vi "Next Message (No Metrics).vi"(8 "error in (no error)":errorcluster, 9 "Timeout ms (-1)":i32=-1, 11 "Module in":refnum<class "Module.lvclass">) -> (0 "error out":errorcluster, 1 "Data":variant, 2 "ID":string, 3 "Module out":refnum<class "Module.lvclass">)   [LabVIEW 2020, in "Volatus.lvlib" / "Module.lvclass"]
uses:
  Module.lvclass
  Module.lvclass/Module.ctl
  MessageQ/MessageQ.lvclass/MessageQ.ctl
  Module Status Update.ctl
  MessageQ/MessageQ.lvclass
  State.ctl
  Module Substatus.ctl
  Metric Update.ctl
  Launch Nested Message.ctl
  VolatusConfig/VolatusConfigElement/VolatusConfigElement.lvclass
  LastAck.ctl
  Update Metric.vi
  Parent Q.vi
  MessageQ/Is Null.vi
  MessageQ/Send.vi
  Volatus.lvlib
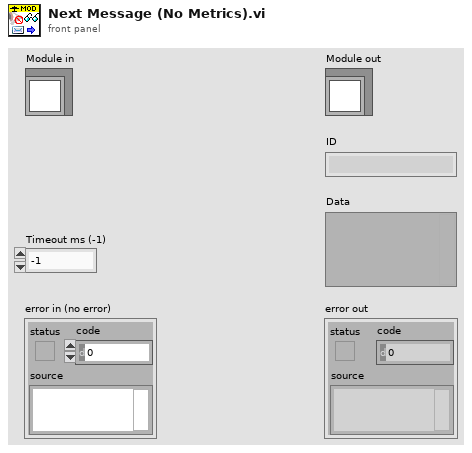
[diagram p1: front panel]
types:
  T1 = typedef "Volatus.lvlib/Module Status Update.ctl" = cluster{"MessageQ":refnum<class "MessageQ.lvclass">, "State":T2, "Hierarchy":string[], "Forwarded":bool}
  T2 = typedef "Volatus.lvlib/Module.lvclass/State.ctl" = enum16{"Unknown", "Launched", "Starting", "Running", "Stopping", "Stopped", "Error - Starting", "Error - Run", "Error - Stopping"}
  T3 = typedef "Volatus.lvlib/Module Substatus.ctl" = cluster{"Hierarchy":string[], "Name":string, "Status":string}
  T4 = typedef "Volatus.lvlib/Metric Update.ctl" = cluster{"Hierarchy":string[], "Name":string, "Value":dbl}
  T5 = typedef "Volatus.lvlib/Launch Nested Message.ctl" = cluster{"Module":refnum<class "Module.lvclass">, "Config":refnum<class "VolatusConfigElement.lvclass">}
  T6 = typedef "Volatus.lvlib/Module.lvclass/LastAck.ctl" = cluster{"Module":refnum<class "Module.lvclass">}
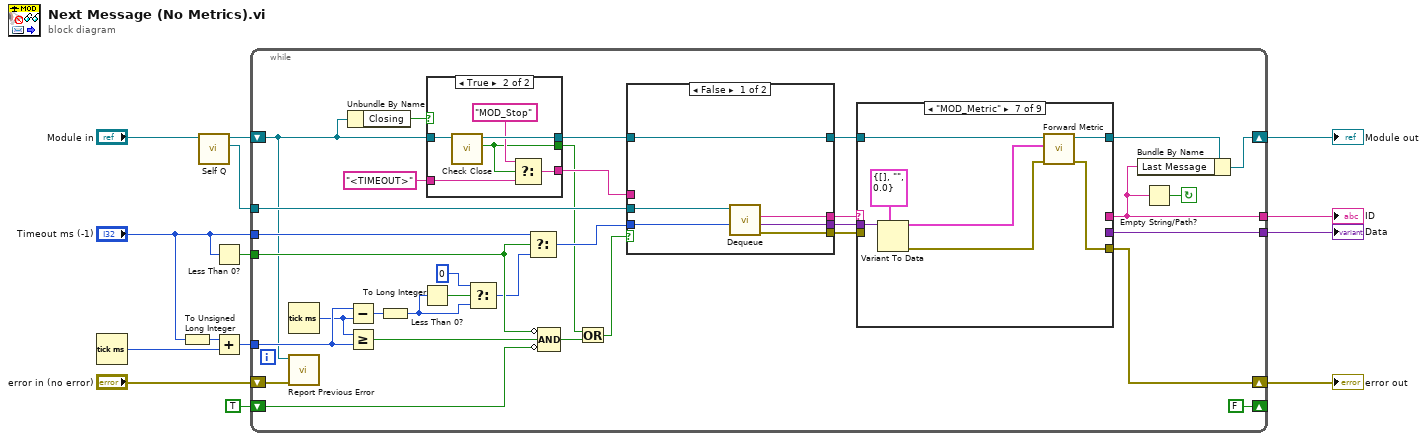
[diagram p0: block diagram]
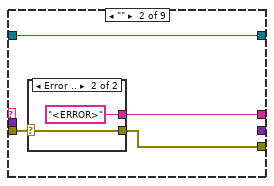
[diagram p5: hidden frame]
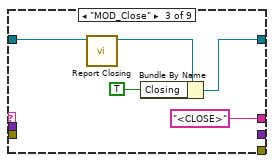
[diagram p7: hidden frame]
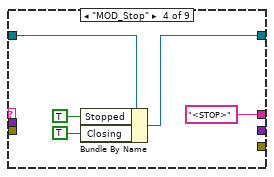
[diagram p8: hidden frame]
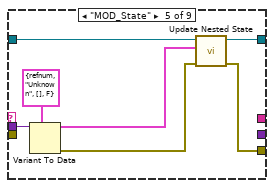
[diagram p9: hidden frame]
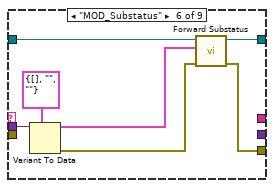
[diagram p10: hidden frame]
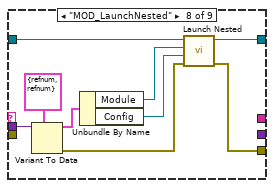
[diagram p11: hidden frame]
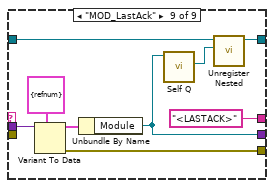
[diagram p12: hidden frame]
diagram:
  n1 = Tick Count (ms)() -> (millisecond timer value=w11:u32)
  n2 = To Unsigned Long Integer(number="Timeout ms (-1)") -> (unsigned 32bit integer=w10:u32)
  n3 = call "Self Q.vi"("Module in"="Module in") -> ("Self Q"=w12:refnum<class "MessageQ.lvclass">, "Module out"=w13:refnum<class "Module.lvclass">)  [unwired: 9 in]
  n4 = Less Than 0?(x="Timeout ms (-1)") -> (x < 0?=w6:bool)
  n5 = Add(x=w10, y=w11) -> (x+y=w9:u32)
  n6 = while {
    shift-right: [w31] -> w1
    shift-left: w13 -> [w15]
    tunnel: w12 -> [w46]
    tunnel: w9 -> [w37]
    tunnel: [w33] -> w3
    tunnel: [w41] -> w8
    tunnel: "Timeout ms (-1)" -> [w39]
    tunnel: w6 -> [w29]
    shift-right: [w34] -> w4
    shift-left: "error in (no error)" -> [w47]
    shift-right: [FALSE] -> _
    shift-left: TRUE -> [w27]
    stop <- w40 continue-if-true
    n7 = Tick Count (ms)() -> (millisecond timer value=w36:u32)
    n8 = call "Report Previous Error.vi"("error in (no error)"=w47, "Module in"=w15) -> ()  [unwired: 8 in, 2 out]
    n9 = Unbundle By Name(w15) -> ("Closing"=w22:bool)
    n10 = Subtract(x=w37, y=w36) -> (x-y=w45:u32)
    n11 = Greater Or Equal?(x=w36, y=w37) -> (x >= y?=w35:bool)
    n12 = To Long Integer(number=w45) -> (32bit integer=w24:i32)
    n13 = Less Than 0?(x=w24) -> (x < 0?=w26:bool)
    n14 = case shown="True" w22 {
      tunnel: w15 -> [w49 w55]
      tunnel: [w49 w54] -> w17
      tunnel: "<TIMEOUT>" ("ID") -> [w48 w53]
      tunnel: [w48 w51] -> w20
      tunnel: [_ w50] -> w18
      frame False {
      }
      frame True {
        n15 = call "Check Close.vi"("Module in"=w55) -> ("Stop"=w50:bool, "Module out"=w54:refnum<class "Module.lvclass">)  [unwired: 8 in, 1 out]
        n16 = Select(t="MOD_Stop", s=w50, f=w53) -> (s? t:f=w51:string)
      }
    }
    n17 = Select(t=0 ("32bit integer"), s=w26, f=w24) -> (s? t:f=w23:i32)
    n18 = Select(t=w39, s=w29, f=w23) -> (s? t:f=w38:i32)
    n19 = Compound Arithmetic op=AND(invert w29, w35, invert w27) -> (w30:bool)
    n20 = Or(x=w18, y=w30) -> (x .or. y?=w19:bool)
    n21 = case shown="False" w19 {
      tunnel: w46 -> [w60 _]
      tunnel: [w59 w63] -> w44
      tunnel: [w58 _] -> w43
      tunnel: [w61 _] -> w42
      tunnel: w38 -> [w57 _]
      tunnel: w20 -> [_ w63]
      tunnel: w17 -> [w56 w62]
      tunnel: [w56 w62] -> w16
      frame False {
        n22 = call "Dequeue.vi"("Timeout ms (-1)"=w57, "MessageQ in"=w60) -> ("error out"=w61:errorcluster, "Data"=w58:variant, "ID"=w59:string)  [unwired: 6 in, 1 out]
      }
      frame True {
      }
    }
    n23 = case shown="\"MOD_Metric\"" w44 {
      selector: w44 -> [w66 _ _ _ _ _ _ _ _]
      tunnel: w43 -> [w64 _ _ _ w89 w96 w103 w112 w121]
      tunnel: w42 -> [_ w68 _ _ _ _ _ _ _]
      tunnel: w16 -> [w65 w70 w77 w81 w87 w94 w101 w109 w115]
      tunnel: [w65 w70 w75 w80 w86 w93 w100 w108 w117] -> w32
      tunnel: [w66 w69 "<CLOSE>" "<STOP>" _ _ _ _ "<LASTACK>"] -> w33
      tunnel: [w64 _ _ _ _ _ _ _ w114] -> w41
      tunnel: [_ w67 _ _ w85 w92 w99 w104 w113] -> w34
      frame Default {
      }
      frame "" {
        n24 = case shown="Error .." w68 {
          selector: w68 -> [_ w71]
          tunnel: [_ "<ERROR>"] -> w69
          tunnel: [_ w71] -> w67
          frame No Error {
          }
          frame Error {
          }
        }
      }
      frame "MOD_Close" {
        n25 = call "Report Closing.vi"("Module in"=w77) -> ("Module out"=w73:refnum<class "Module.lvclass">)  [unwired: 9 in, 1 out]
        n26 = Bundle By Name(cluster=w73, "Closing"=TRUE) -> (w75:refnum<class "Module.lvclass">)
      }
      frame "MOD_Stop" {
        n27 = Bundle By Name(cluster=w81, "Stopped"=TRUE, "Closing"=TRUE) -> (w80:refnum<class "Module.lvclass">)
      }
      frame "MOD_State" {
        n28 = Variant To Data(type=T1 {"MessageQ"=refnum, "State"=enum."Unknown", "Hierarchy"=[], "Forwarded"=FALSE} ("Nested State Data"), Variant=w89) -> (data=w83:T1, error out=w84:errorcluster)  [unwired: 1 in]
        n29 = call "Update Nested State.vi"("error in (no error)"=w84, "Module Status"=w83, "Module in"=w87) -> ("error out"=w85:errorcluster, "Module out"=w86:refnum<class "Module.lvclass">)  [unwired: 7 in]
      }
      frame "MOD_Substatus" {
        n30 = Variant To Data(type=T3 {"Hierarchy"=[], "Name"="", "Status"=""} ("Nested State Data"), Variant=w96) -> (data=w90:T3, error out=w91:errorcluster)  [unwired: 1 in]
        n31 = call "Forward Substatus.vi"("error in (no error)"=w91, "Module Substatus"=w90, "Module in"=w94) -> ("error out"=w92:errorcluster, "Module out"=w93:refnum<class "Module.lvclass">)  [unwired: 7 in]
      }
      frame "MOD_Metric" {
        n32 = Variant To Data(type=T4 {"Hierarchy"=[], "Name"="", "Value"=0.0} ("Nested State Data"), Variant=w103) -> (data=w97:T4, error out=w98:errorcluster)  [unwired: 1 in]
        n33 = call "Forward Metric.vi"("error in (no error)"=w98, "Metric Update"=w97, "Module in"=w101) -> ("error out"=w99:errorcluster, "Module out"=w100:refnum<class "Module.lvclass">)  [unwired: 7 in]
      }
      frame "MOD_LaunchNested" {
        n34 = Variant To Data(type=T5 {"Module"=refnum, "Config"=refnum} ("Launch Nested Message"), Variant=w112) -> (data=w110:T5, error out=w105:errorcluster)  [unwired: 1 in]
        n35 = Unbundle By Name(w110) -> ("Module"=w107:refnum<class "Module.lvclass">, "Config"=w106:refnum<class "VolatusConfigElement.lvclass">)
        n36 = call "Launch Nested.vi"("error in (no error)"=w105, "Config Element"=w106, "Nested Module"=w107, "Parent in"=w109) -> ("error out"=w104:errorcluster, "Parent out"=w108:refnum<class "Module.lvclass">)  [unwired: 5 in, 1 out]
      }
      frame "MOD_LastAck" {
        n37 = Variant To Data(type=T6 {"Module"=refnum} ("LastAck"), Variant=w121) -> (data=w119:T6, error out=w113:errorcluster)  [unwired: 1 in]
        n38 = Unbundle By Name(w119) -> ("Module"=w114:refnum<class "Module.lvclass">)
        n39 = call "Self Q.vi"("Module in"=w114) -> ("Self Q"=w118:refnum<class "MessageQ.lvclass">)  [unwired: 9 in, 1 out]
        n40 = call "Unregister Nested.vi"("MessageQ"=w118, "Module in"=w115) -> ("Module out"=w117:refnum<class "Module.lvclass">)  [unwired: 8 in, 1 out]
      }
    }
    n41 = Bundle By Name(cluster=w32, "Last Message"=w33) -> (w31:refnum<class "Module.lvclass">)
    n42 = Empty String/Path?(string/path=w33) -> (empty?=w40:bool)
  }
  "error out" <- w4
  "Module out" <- w1
  "ID" <- w3
  "Data" <- w8
